vi "Parse-element.vi"(8 "error in (no error)":errorcluster, 10 "String in":string, 11 "JumpAbs in":refnum<class "JumpAbs.lvclass">) -> (0 "error out":errorcluster, 1 "Valid element?":bool, 2 "Remaining string":string, 3 "JumpAbs out":refnum<class "JumpAbs.lvclass">)   [LabVIEW 2013, in "HardwareCharacterization.lvlib" / "JumpAbs.lvclass"]
uses:
  JumpAbs.lvclass
  JumpAbs.lvclass/JumpAbs.ctl
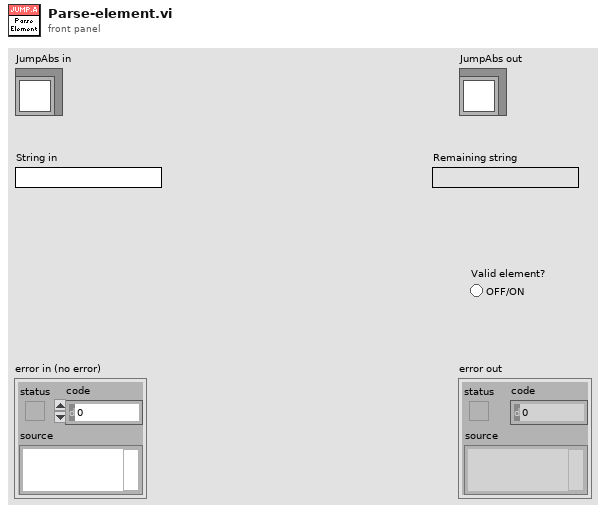
[diagram p1: front panel]
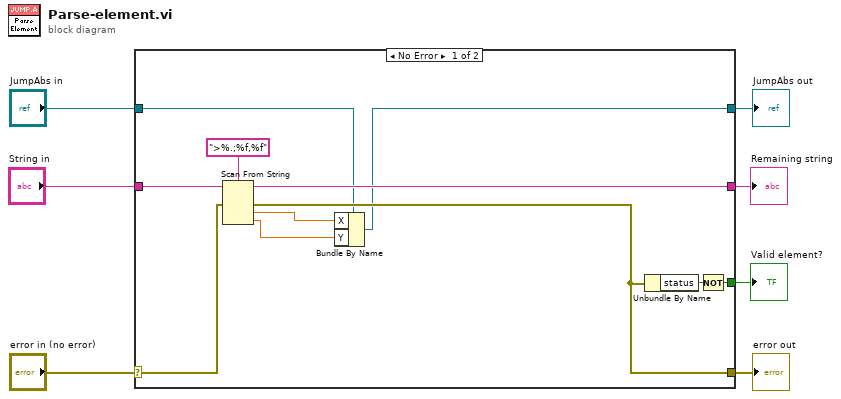
[diagram p0: block diagram]
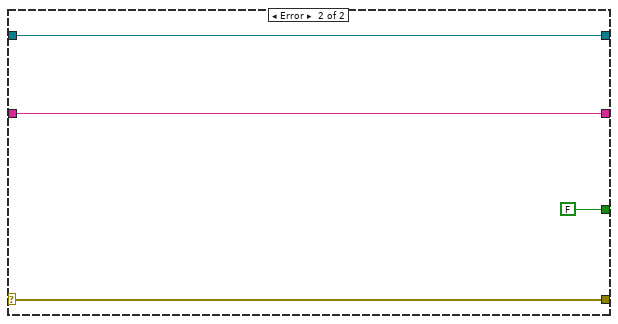
[diagram p2: hidden frame]
diagram:
  n1 = case shown="No Error" "error in (no error)" {
    selector: "error in (no error)" -> [w17 w22]
    tunnel: [w14 w22] -> w6
    tunnel: [w10 w21] -> w4
    tunnel: "JumpAbs in" -> [w11 w21]
    tunnel: "String in" -> [w18 w20]
    tunnel: [w15 w20] -> w2
    tunnel: [w12 FALSE] -> w1
    frame No Error {
      n2 = Scan From String(format string=">%.;%f,%f", input string=w18, error in=w17) -> (remaining string=w15:string, error out=w14:errorcluster, output 1=w9:dbl, output 2=w8:dbl)  [unwired: 3 in, 1 out]
      n3 = Bundle By Name(cluster=w11, "X"=w9, "Y"=w8) -> (w10:refnum<class "JumpAbs.lvclass">)
      n4 = Unbundle By Name(w14) -> ("status"=w13:bool)
      n5 = Not(x=w13) -> (.not. x?=w12:bool)
    }
    frame Error {
    }
  }
  "error out" <- w6
  "JumpAbs out" <- w4
  "Valid element?" <- w1
  "Remaining string" <- w2
